vi "init_ccd_sbig_2_camera.vi"(4 "Step size":dbl, 5 "Scan Prefix":string="test", 6 "Max nm":dbl, 7 "Min nm":dbl, 8 "Exposure Time":dbl, 9 "Scan Directory":string="Peter_ferguson\\Tcal\\scans\\") -> (2 "Working Directory":path)   [LabVIEW 2018]
uses:
  <vilib>/Utility/sysdir.llb/System Directory Type.ctl
panel:
  in  "CCD control name":string="CCDautomation2camera.exe"
  in  "CCD control Directory":string="\\Peter_ferguson\\Tcal\\Labview_Code\\Other_Libraries\\MoCoAuto\\"
  out "Commands Sent":string
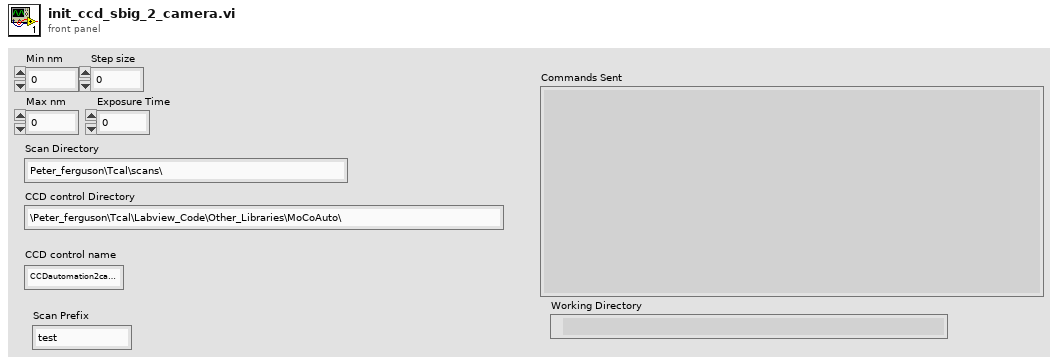
[diagram p1: front panel]
types:
  T1 = enum16{"open", "replace", "create", "open or create", "replace or create", "replace or create with confirmation"}
  T2 = typedef "System Directory Type.ctl" = i32
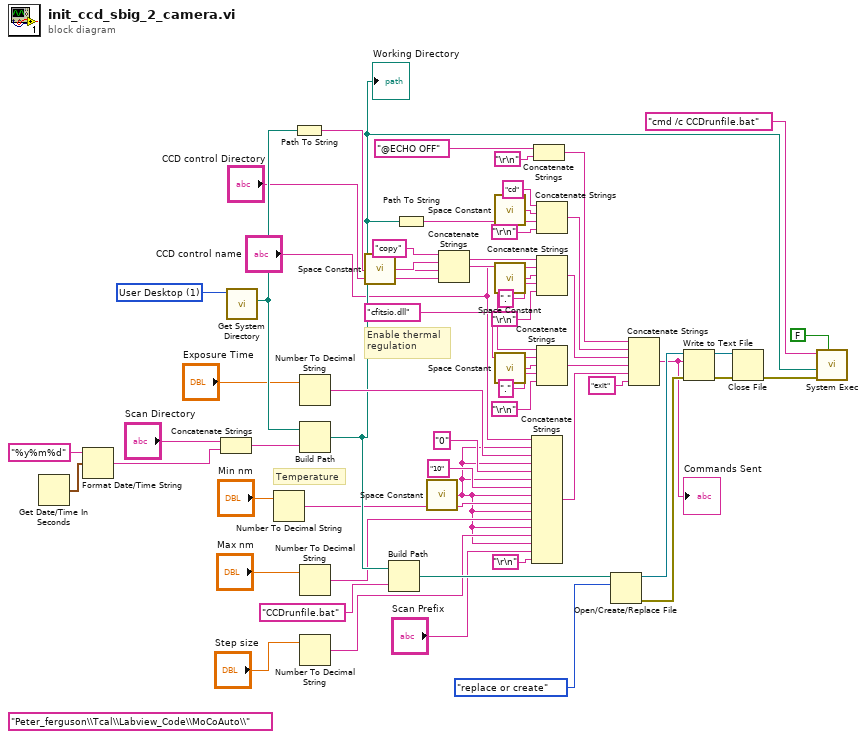
[diagram p0: block diagram]
diagram:
  (unwired) "Peter_ferguson\\Tcal\\Labview_Code\\MoCoAuto\\" ("string")
  w55 = T2 1 items=["User Home"=0, "User Desktop"=1, "User Documents"=2, "User Application Data"=3, "User Preferences"=4, "User Temporary"=5, "Public Documents"=6, "Public Application Data"=7, "Public Preferences"=8, "Public Cache"=13, "System Core Libraries"=9, "System Installed Libraries"=10, "Application Files"=11, "Boot Volume Root"=12] ("system directory type")
  # "Temperature"
  # "Enable thermal regulation"
  n1 = Get Date/Time In Seconds() -> (seconds since 1Jan1904=w57:timestamp)
  n2 = Format Date/Time String(time format string (%c)="%y%m%d", seconds (now)=w57) -> (date/time string=w53:string)  [unwired: 1 in]
  n3 = Concatenate Strings("Scan Directory", w53) -> (w52:string)
  n4 = call <vilib>:"Get System Directory.vi"("system directory type"=w55) -> ("system directory"=w51:path)  [unwired: 10 in]
  n5 = Number To Decimal String(number="Min nm") -> (decimal integer string=w8:string)  [unwired: 1 in]
  n6 = Path To String(path=w51) -> (string=w42:string)
  n7 = Number To Decimal String(number="Exposure Time") -> (decimal integer string=w28:string)  [unwired: 1 in]
  n8 = Build Path(base path=w51, name or relative path=w52) -> (appended path=w15:path)
  "Working Directory" <- w15
  n9 = Number To Decimal String(number="Max nm") -> (decimal integer string=w7:string)  [unwired: 1 in]
  n10 = Number To Decimal String(number="Step size") -> (decimal integer string=w6:string)  [unwired: 1 in]
  n11 = call <vilib>:"Space Constant.vi"() -> ("String"=w43:string)
  n12 = Build Path(base path=w15, name or relative path="CCDrunfile.bat") -> (appended path=w22:path)
  n13 = Path To String(path=w15) -> (string=w46:string)
  n14 = call <vilib>:"Space Constant.vi"() -> ("String"=w5:string)
  n15 = Concatenate Strings("copy", w43, w42, "CCD control Directory") -> (w35:string)
  n16 = call <vilib>:"Space Constant.vi"() -> ("String"=w47:string)
  n17 = call <vilib>:"Space Constant.vi"() -> ("String"=w39:string)
  n18 = call <vilib>:"Space Constant.vi"() -> ("String"=w33:string)
  n19 = Concatenate Strings("CCD control name", w5, w28, w5, "0" ("string"), w5, "10" ("string"), w5, w8, w5, w7, w5, w6, w5, "Scan Prefix", "\r\n") -> (w11:string)
  n20 = Concatenate Strings("@ECHO OFF" ("string"), "\r\n") -> (w41:string)
  n21 = Concatenate Strings("cd" ("string"), w47, w46, "\r\n") -> (w40:string)
  n22 = Concatenate Strings(w35, "CCD control name", w39, "." ("string"), "\r\n") -> (w36:string)
  n23 = Concatenate Strings(w35, "cfitsio.dll" ("string"), w33, "." ("string"), "\r\n") -> (w30:string)
  n24 = Open/Create/Replace File(file path (use dialog)=w22, operation (0:open)=T1."replace or create") -> (refnum out=w19:refnum<file>, error out=w18:errorcluster)  [unwired: 4 in, 1 out]
  n25 = Concatenate Strings(w41, w40, w36, w30, w11, "exit" ("string")) -> (w16:string)
  "Commands Sent" <- w16
  n26 = Write to Text File(file (use dialog)=w19, text=w16, error in=w18) -> (refnum out=w20:refnum<file>, error out=w17:errorcluster)  [unwired: 1 in, 1 out]
  n27 = Close File(refnum=w20, error in=w17) -> (error out=w12:errorcluster)  [unwired: 1 out]
  n28 = call <vilib>:"System Exec.vi"("wait until completion? (T)"=FALSE, "error in (no error)"=w12, "working directory"=w15, "command line"="cmd /c CCDrunfile.bat") -> ()  [unwired: 4 in, 4 out]
